vi "A - write log line_no_Regexp V2.vi"(6 "file is new?":bool=TRUE, 9 "temperature boxes":T1={"LTC21 Address"="GPIB0::15::INSTR", "ITC503 Address"="GPIB0::24::INSTR", "ITC temperature"=299.2, "ITC set temperature"=295.0, "LTC temperature"=0.0, "heater"=0.0, "gas flow"=90.0, "P"=10.0, "D"=1.0, "I"=3.0, "ITC state"="X0A1C2S00H1L0\r", "nonzero temperature"=0.0, "Field (T)"=0.0, "LakeShore340"="", "LS340 Adress"=0, "Sample Temperature Source"=enum."read T <- LakeShore 340", "Neocera sensor"=1, "Magnetic Field Source"=enum."None", "field scale"=0.6578903516080653} {"field scale" format="%#_16g"}, 11 "file Path":path) -> ()   [LabVIEW 2015]
uses:
  state.ctl
  Sample_Temperature_Source_Control.ctl
  <vilib>/Utility/file.llb/Write To Spreadsheet File (string).vi
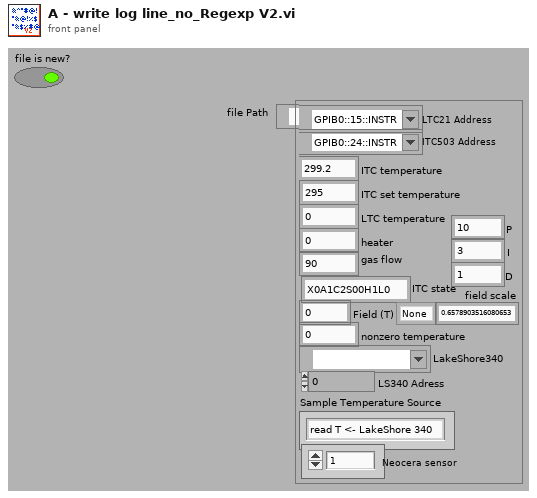
[diagram p1: front panel]
types:
  T1 = typedef "state.ctl" = cluster{"LTC21 Address":refnum<visa-resource-name>, "ITC503 Address":refnum<visa-resource-name>, "ITC temperature":dbl, "ITC set temperature":dbl, "LTC temperature":dbl, "heater":dbl, "gas flow":dbl, "P":dbl, "D":dbl, "I":dbl, "ITC state":string, "nonzero temperature":dbl, "Field (T)":dbl, "LakeShore340":refnum<visa-resource-name>, "LS340 Adress":i16, "Sample Temperature Source":T2, "Neocera sensor":i32, "Magnetic Field Source":enum16{"None", "20T", "DTM"}, "field scale":dbl}
  T2 = typedef "Sample_Temperature_Source_Control.ctl" = enum16{"read T <- LakeShore 340", "read T <- Neocera"}
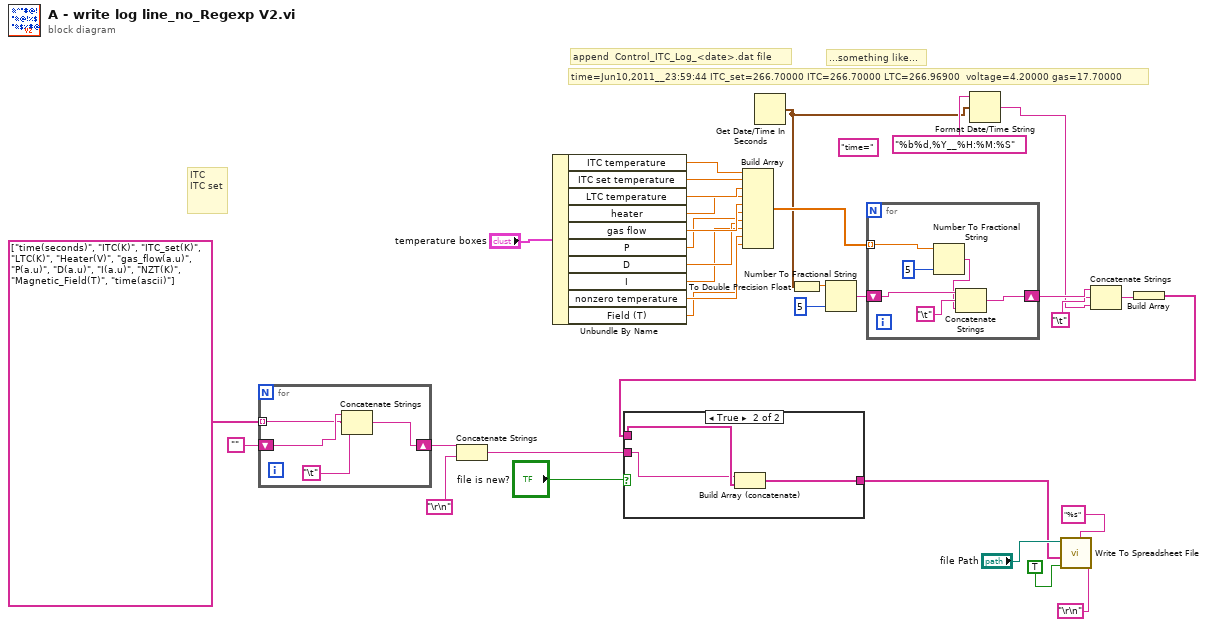
[diagram p0: block diagram]
diagram:
  (unwired) "time=" ("string")
  # "ITC\nITC set"
  # "...something like..."
  # "time=Jun10,2011__23:59:44\tITC_set=266.70000\tITC=266.70000\tLTC=266.96900\t\tvoltage=4.20000\tgas=17.70000"
  # "append  Control_ITC_Log_<date>.dat file"
  n1 = for {
    tunnel: string[] ["time(seconds)", "ITC(K)", "ITC_set(K)", "LTC(K)", "Heater(V)", "gas_flow(a.u)", "P(a.u)", "D(a.u)", "I(a.u)", "NZT(K)", "Magnetic_Field(T)", "time(ascii)"] -> [w36] mode=indexing
    shift-right: [w34] -> w14
    shift-left: "" -> [w37]
    n2 = Concatenate Strings(w37, w36, "\t") -> (w34:string)
  }
  n3 = Concatenate Strings(w14, "\r\n") -> (w12:string)
  n4 = Unbundle By Name("temperature boxes") -> ("ITC temperature"=w10:dbl, "ITC set temperature"=w9:dbl, "LTC temperature"=w8:dbl, "heater"=w7:dbl, "gas flow"=w6:dbl, "P"=w5:dbl, "D"=w4:dbl, "I"=w3:dbl, "nonzero temperature"=w2:dbl, "Field (T)"=w1:dbl)
  n5 = Build Array(w10, w9, w8, w7, w6, w5, w4, w3, w2, w1) -> (w27:dbl[])
  n6 = Get Date/Time In Seconds() -> (seconds since 1Jan1904=w22:timestamp)
  n7 = To Double Precision Float(number=w22) -> (double precision float=w25:dbl)
  n8 = Number To Fractional String(number=w25, precision (6)=i16 5 ("width (-)")) -> (F-format string=w24:string)  [unwired: 2 in]
  n9 = for {
    tunnel: w27 -> [w43] mode=indexing
    shift-right: [w41] -> w23
    shift-left: w24 -> [w40]
    n10 = Number To Fractional String(number=w43, precision (6)=i16 5 ("width (-)")) -> (F-format string=w38:string)  [unwired: 2 in]
    n11 = Concatenate Strings(w40, "\t", w38) -> (w41:string)
  }
  n12 = Format Date/Time String(time format string (%c)="%b%d,%Y__%H:%M:%S", seconds (now)=w22) -> (date/time string=w20:string)  [unwired: 1 in]
  n13 = Concatenate Strings(w23, "\t", w20) -> (w19:string)
  n14 = Build Array(w19) -> (w18:string[])
  n15 = case shown="True" "file is new?" {
    tunnel: [w44 w47] -> w11
    tunnel: w18 -> [w44 w46]
    tunnel: w12 -> [_ w45]
    frame False {
    }
    frame True {
      n16 = Build Array (concatenate)(w45, w46) -> (w47:string[])
    }
  }
  n17 = call-poly <vilib>:"Write To Spreadsheet File.vi"("delimiter (\\t)"="\r\n", "format (%s)"="%s", "append to file? (new file:F)"=TRUE, "1D data"=w11, "file path (dialog if empty)"="file Path") -> ()  [unwired: 3 in, 1 out]
